vi "Get Formatted Buffer.vi"(8 "error in (no error)":errorcluster, 11 "Measure in":refnum<class "Measure.lvclass">) -> (0 "error out":errorcluster, 2 "Buffer Name":string, 3 "Measure out":refnum<class "Measure.lvclass">)   [LabVIEW 2023, in "HAF.lvlib" / "Measure.lvclass"]
doc: "Returns the name of the Buffer to be used by the instrument to save the measured value. If the Buffer hasn't been configured, it will use either a Default value, if supported, or return an empty name and no buffer will be used."
uses:
  Measure.lvclass
  Measure.lvclass/Measure.ctl
  Driver/Driver.lvclass
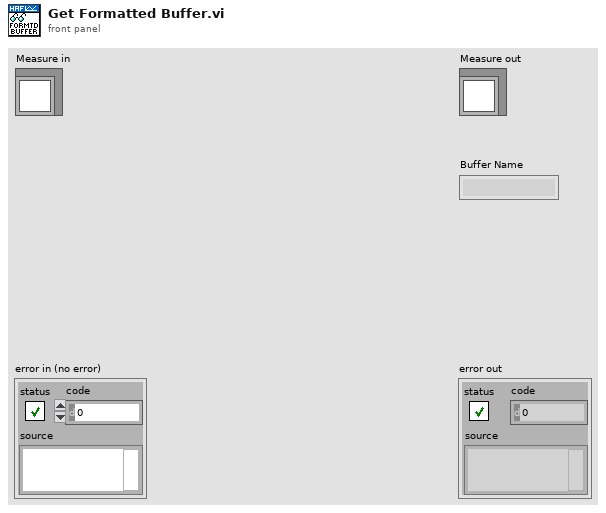
[diagram p1: front panel]
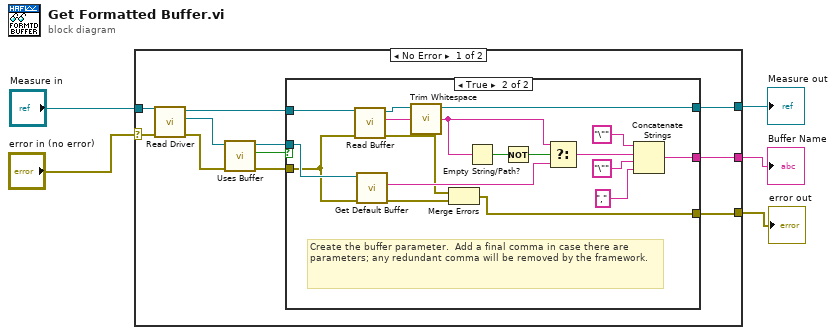
[diagram p0: block diagram]
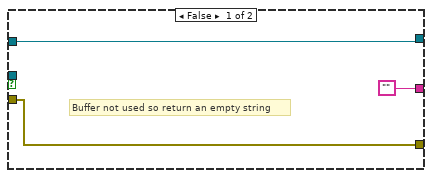
[diagram p2: hidden frame]
diagram:
  n1 = case shown="No Error" "error in (no error)" {
    selector: "error in (no error)" -> [w15 w37]
    tunnel: [w7 w38] -> w3
    tunnel: "Measure in" -> [w16 w38]
    tunnel: [w8 _] -> w2
    tunnel: [w6 w37] -> w1
    frame No Error {
      n2 = call-dynamic "Read Driver.vi"("error in (no error)"=w15, "WriteCommand in"=w16) -> ("error out"=w13:errorcluster, "Driver"=w14:refnum<class "Driver.lvclass">, "WriteCommand out"=w9:refnum<class "Measure.lvclass">)  [unwired: 7 in]
      n3 = call-dynamic "Uses Buffer.vi"("error in (no error)"=w13, "Driver in"=w14) -> ("error out"=w10:errorcluster, "Uses Buffer"=w12:bool, "Driver out"=w11:refnum<class "Driver.lvclass">)  [unwired: 7 in]
      n4 = case shown="True" w12 {
        tunnel: w11 -> [_ w34]
        tunnel: w10 -> [w18 w33]
        tunnel: w9 -> [w19 w36]
        tunnel: ["" w22] -> w8
        tunnel: [w19 w21] -> w7
        tunnel: [w18 w20] -> w6
        frame False {
          # "Buffer not used so return an empty string"
        }
        frame True {
          # "Create the buffer parameter.  Add a final comma in case there are parameters; any redundant comma will be removed by the framework."
          n5 = call-dynamic "Read Buffer.vi"("error in (no error)"=w33, "Measure in"=w36) -> ("error out"=w28:errorcluster, "Buffer"=w35:string, "Measure out"=w21:refnum<class "Measure.lvclass">)  [unwired: 7 in]
          n6 = call-dynamic "Get Default Buffer.vi"("error in (no error)"=w33, "Driver in"=w34) -> ("error out"=w27:errorcluster, "Buffer"=w29:string)  [unwired: 7 in, 1 out]
          n7 = call <vilib>:"Trim Whitespace.vi"("string"=w35) -> ("trimmed string"=w30:string)  [unwired: 1 in]
          n8 = Merge Errors(w28, w27) -> (w20:errorcluster)
          n9 = Empty String/Path?(string/path=w30) -> (empty?=w32:bool)
          n10 = Not(x=w32) -> (.not. x?=w31:bool)
          n11 = Select(t=w30, s=w31, f=w29) -> (s? t:f=w26:string)
          n12 = Concatenate Strings("\"" ("string"), w26, "\"" ("string"), "," ("string")) -> (w22:string)
        }
      }
    }
    frame Error {
    }
  }
  "error out" <- w1
  "Measure out" <- w3
  "Buffer Name" <- w2
